vi "example_01_build_interface.vi"   [LabVIEW 2015, in "lv-builder-l3.lvlib"]
uses:
  lv-builder-l3.lvlib
  <userlib>/antonio-alexander/lv-build/lv-build-interface/lv-build-interface.lvlib
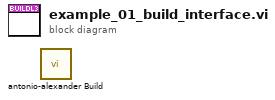
[diagram p0: block diagram]
diagram:
  n1 = call "antonio-alexander Build.vi"() -> ()  [unwired: 11 in, 1 out]
